vi "Eval.Python.vi"(0 "input":string) -> ()   [LabVIEW 2014]
uses:
  python27.dll
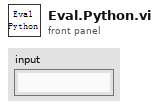
[diagram p1: front panel]
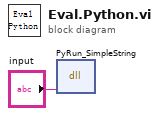
[diagram p0: block diagram]
diagram:
  n1 = dll-call lib="python27.dll" fn="PyRun_SimpleString"("code"="input") -> ()  [unwired: 5 in, 2 out]
